vi "Untitled 1.vi"() -> ()   [LabVIEW 2026]
panel:
  out "output array":bool[](array[boolean])
  in  "Player 1 Output":bool[][](array[boolean])=[[FALSE, FALSE, FALSE, FALSE]]
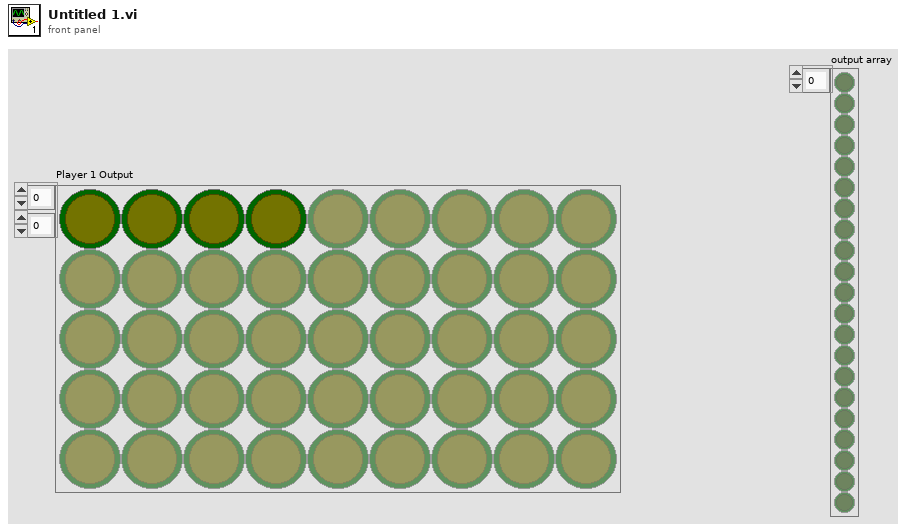
[diagram p1: front panel]
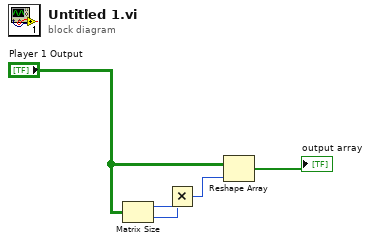
[diagram p0: block diagram]
diagram:
  n1 = Matrix Size(0:"Player 1 Output") -> (1:w5:i32, 2:w4:i32)
  n2 = Multiply(x=w5, y=w4) -> (x*y=w3:i32)
  n3 = Reshape Array("Player 1 Output", w3) -> (→"output array":bool[])
